vi "Wind Turbine 2021.vi"() -> (0 "DAQ Error":errorcluster)   [LabVIEW 2020]
doc: "Use this plug-in with the Nathan 7609 data acquisition system"
uses:
  <vilib>/Instr/_visa.llb/VISA Find Search Mode.ctl
  Globals/Meas_global.vi
panel:
  # "Ch 0  Motor RPM\nCh1   Motor Current (A)\nCh2   Photo darlington (V)\nCh3   Duty (-1....1)"
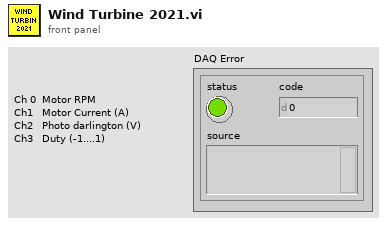
[diagram p1: front panel]
types:
  T1 = typedef "Analysis_info_cluster.ctl" = cluster{"Colour":u32, "Inst type":T2, "Inst name":string, "Symbol":string, "Code name":string, "Extra Info":string, "Inst Array":T3, "Extra Titles":string[], "Extra Values":string[], "U":dbl, "u^2":dbl, "u^3":dbl, "u^4":dbl, "Skew_u":dbl, "Kurt_u":dbl, "Sd Error in Mean":dbl, "% u'/U":dbl, "X":dbl, "Y":dbl, "Z":dbl, "Timescale integral Estimate":dbl, "Sd Error in Variance":dbl, "Calib File":path, "Calib Constants":dbl[], "Output Position":bool, "Stats":enum16{"None", "Basic", "Full"}, "Av Sampling Rate":dbl, "Av No of Samples":dbl, "Total Meas Time (s)":dbl, "ADAM Ch Name":string, "Max value":dbl, "Min value":dbl, "Req Sample Rate Hz":dbl, "Sync Delay Time (s)":dbl, "Ch No":i16, "Device":string, "Use Latest Calib":bool, "Port":string, "Metadata Ch Names":string[], "Metadata Ch Values":string[], "Label":string}
  T2 = typedef "Inst_type.ctl" = enum16{"Raw voltage", "Raw with zero offsetting", "Propeller anemometer", "Pressure Transducer", "Pitot-static tube", "Hot wire", "Cross wire 1", "Cross wire 2", "Generic Linear", "Generic Polynomial", "Generic BackPoly", "Fast FID", "Thermocouple", "Cold wire", "Pulsed Wire", "LDA Vel", "LDA Tran time", "LDA Arr time", "Microphone"}
  T3 = typedef "Instrument_Array.ctl" = enum16{"PWA", "LDA", "Analogue"}
  T4 = typedef "Setup.ctl" = enum16{"Run Program", "Show Setup", "Save Current Setup", "Setup Front Panel"}
  T5 = typedef "Device ID port info.ctl" = cluster{"Ch No":i16[], "Req Sampling Rate":dbl[], "Port":string, "Index":i32[]}
  T6 = typedef "VISA Find Search Mode.ctl" = u32
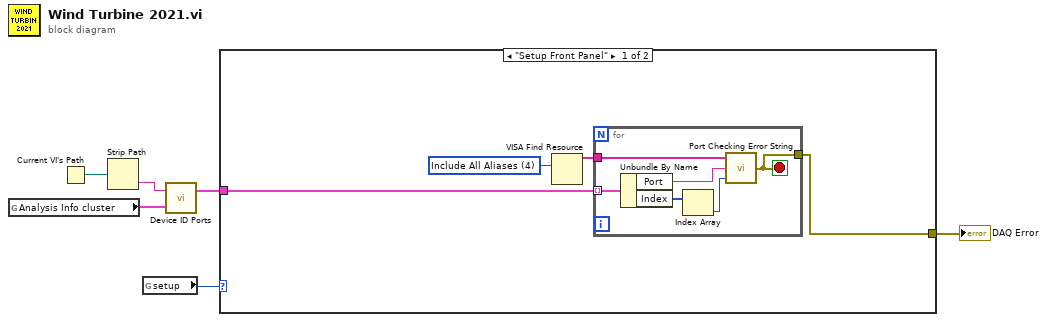
[diagram p0: block diagram]
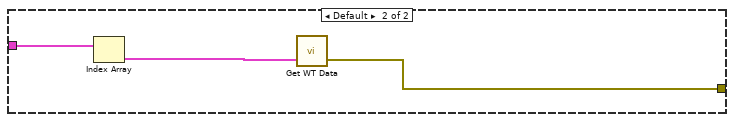
[diagram p2: hidden frame]
diagram:
  n1 = global read "Meas_global.vi" "Analysis Info cluster"() -> (w5:T1[])
  n2 = Current VI's Path() -> (path=w6:path)
  n3 = Strip Path(path=w6) -> (name=w4:string)  [unwired: 1 out]
  n4 = global read "Meas_global.vi" "setup"() -> (w1:T4)
  n5 = call "Device ID Ports.vi"("Analysis Info cluster"=w5, "Device ID"=w4) -> ("Device port info"=w3:T5[])  [unwired: 1 out]
  n6 = case shown="\"Setup Front Panel\"" w1 {
    tunnel: w3 -> [w10 w19]
    tunnel: [w7 w17] -> w2
    frame "Setup Front Panel" {
      w9 = T6 4 items=["Canonical Names Only"=0, "Aliases Only"=1, "Include Matching Aliases"=2, "Include All Aliases"=4] ("Search Mode")
      n7 = VISA Find Resource(10:w9) -> (3:w8:string[])  [unwired: 2 in, 2 out]
      n8 = for {
        tunnel: w10 -> [w16] mode=indexing
        tunnel: w8 -> [w12]
        tunnel: [w11] -> w7
        stop <- w11 stop-if-true
        n9 = Unbundle By Name(w16) -> ("Port"=w13:string, "Index"=w15:i32[])
        n10 = Index Array(array=w15) -> (element=w14:i32)  [unwired: 1 in]
        n11 = call "Port Checking Error String.vi"("Ch Index"=w14, "Port"=w13, "Available Ports"=w12) -> ("error out"=w11:errorcluster)  [unwired: 1 in]
      }
    }
    frame Default {
      n12 = Index Array(array=w19) -> (element=w18:T5)  [unwired: 1 in]
      n13 = call "Get WT Data.vi"("Device Info"=w18) -> ("Error out"=w17:errorcluster)  [unwired: 2 in]
    }
  }
  "DAQ Error" <- w2
